vi "Destroy DAQmx Input Refs.vi"(8 "error in (no error)":errorcluster, 11 "DAQ":refnum<class "DAQ.lvclass">) -> (0 "error out":errorcluster, 3 "DAQ":refnum<class "DAQ.lvclass">)   [LabVIEW 2017, in "DAQ.lvclass"]
doc: "Developed by Kevin Thompson\nkevin@thompsonengineering.net\n\nCopyright 2018-2020\nThompson Engineering, LLC"
uses:
  DAQ.lvclass
  DAQ.lvclass/DAQ.ctl
  DataTypes/TD AI TaskIO.ctl
  DataTypes/TD DI TaskIO.ctl
  Accessors/Get DAQNodes Dict.vi
  Accessors/Get IO Nodes.vi
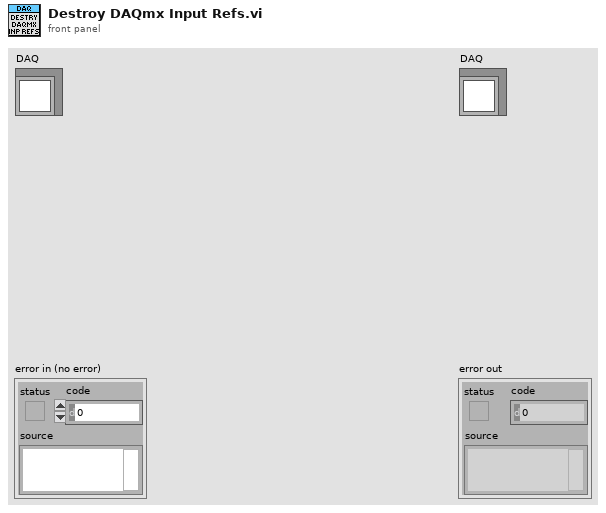
[diagram p1: front panel]
types:
  T1 = typedef "TD Dynamic CVT DVR--ref.ctl" = refnum<data-value>
  T2 = typedef "DAQ.lvclass/TD IO Config Definition--cluster.ctl" = cluster{"DI Config":T3, "DO Config":T6, "AI Config":T8, "AO Config":T14}
  T3 = typedef "DAQ.lvclass/TD DI Config--cluster.ctl" = cluster{"DI Tasks":T4[]}
  T4 = typedef "DAQ.lvclass/TD DI Task--cluster.ctl" = cluster{"DI TaskName":string, "DI Channels":T5[]}
  T5 = typedef "DAQ.lvclass/TD DI Channel--cluster.ctl" = cluster{"DevName":string, "IOName":string, "IOPath":string, "SchemName":string, "logic":enum16{"Lo", "Hi"}, "Index":i32}
  T6 = typedef "DAQ.lvclass/TD DO Config--cluster.ctl" = cluster{"DO Channels":T7[]}
  T7 = typedef "DAQ.lvclass/TD DO Channel--cluster.ctl" = cluster{"DevName":string, "IOName":string, "IOPath":string, "SchemName":string, "logic":enum16{"Lo", "Hi"}, "DAQmx Task":refnum<k21>}
  T8 = typedef "DAQ.lvclass/TD AI Config--cluster.ctl" = cluster{"AI Tasks":T9[]}
  T9 = typedef "DAQ.lvclass/TD AI Task--cluster.ctl" = cluster{"AI TaskName":string, "AI Channels":T10[]}
  T10 = typedef "DAQ.lvclass/TD AI Channel--cluster.ctl" = cluster{"DevName":string, "IOName":string, "IOPath":string, "SchemName":string, "MinValue":dbl, "MaxValue":dbl, "Terminal Configuration":i32, "Index":i32, "Conversion":T11, "AIType":T12, "Force Bridge":T13}
  T11 = typedef "DAQ.lvclass/TD DataValueConversion--cluster.ctl" = cluster{"MaxSignal":dbl, "MinSignal":dbl, "MaxEngUnit":dbl, "MinEngUnit":dbl, "ScaleOffset":dbl, "negate":bool}
  T12 = typedef "DAQ.lvclass/TD AI DAQ Type--enum.ctl" = enum16{"Voltage", "Current", "Strain Gage", "Force Bridge"}
  T13 = typedef "DAQ.lvclass/TD AI Force Bridge--cluster.ctl" = cluster{"bridge information":cluster{"bridge configuration":i32, "voltage excitation source":i32, "voltage excitation value":dbl, "nominal bridge resistance":dbl}, "scaling information":cluster{"first electrical value":dbl, "second electrical value":dbl, "electrical units":i32, "first physical value":dbl, "second physical value":dbl, "physical units":i32}}
  T14 = typedef "DAQ.lvclass/TD AO Config--cluster.ctl" = cluster{"AO Channels":T15[]}
  T15 = typedef "DAQ.lvclass/TD AO Channel--cluster.ctl" = cluster{"DevName":string, "IOName":string, "IOPath":string, "SchemName":string, "Vmin":dbl, "Vmax":dbl, "Conversion":T11, "DAQmx Task":refnum<k21>}
  T16 = typedef "DAQ.lvclass/TD AI TaskIO.ctl" = cluster{"AI TaskName":string, "IONames":string[], "DAQmx AI TaskRef":refnum<k21>}
  T17 = typedef "DAQ.lvclass/TD DI TaskIO.ctl" = cluster{"DI TaskName":string, "IONames":string[], "DAQmxDI TaskRef":refnum<k21>}
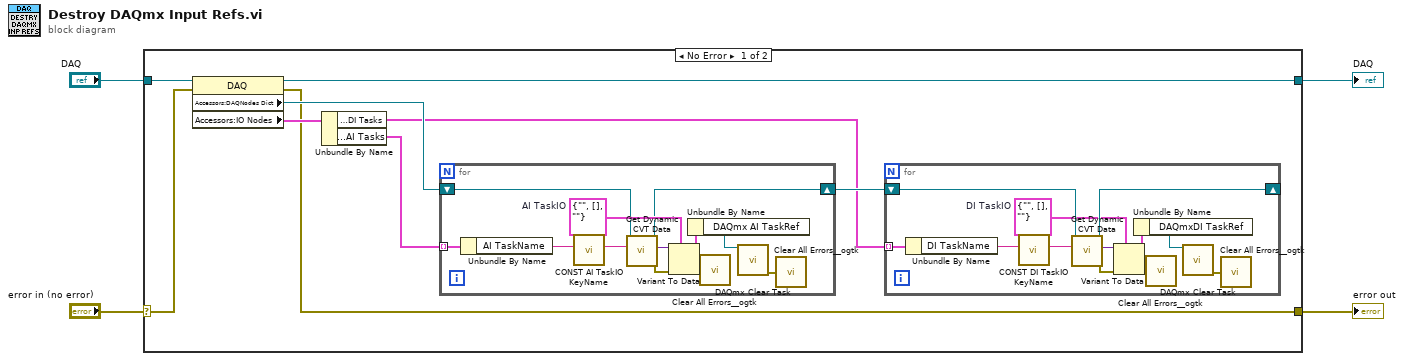
[diagram p0: block diagram]
diagram:
  n1 = case shown="No Error" "error in (no error)" {
    selector: "error in (no error)" -> [w6 w39]
    tunnel: [w5 w39] -> w3
    tunnel: [w12 w38] -> w1
    tunnel: "DAQ" -> [w13 w38]
    frame No Error {
      n2 = property class="DAQ"(reference=w13, error in=w6) -> (reference out=w12:refnum<class "DAQ.lvclass">, error out=w5:errorcluster, "Accessors:DAQNodes Dict"=w9:T1, "Accessors:IO Nodes"=w11:T2)
      n3 = Unbundle By Name(w11) -> ("DI Config.DI Tasks"=w7:T4[], "AI Config.AI Tasks"=w10:T9[])
      n4 = for {
        tunnel: w10 -> [w34] mode=indexing
        shift-right: [w27] -> w8
        shift-left: w9 -> [w28]
        w31 = T16 {"AI TaskName"="", "IONames"=[], "DAQmx AI TaskRef"=""}  # AI TaskIO
        n5 = Unbundle By Name(w34) -> ("AI TaskName"=w33:string)
        n6 = call "CONST AI TaskIO KeyName.vi"("AI TaskName"=w33) -> ("AI TaskIO (KeyName)"=w32:string)  [unwired: 10 in]
        n7 = call <vilib>:"Get Dynamic CVT Data.vi"("DataName"=w32, "dCVT DVR"=w28) -> ("error out"=w37:errorcluster, "value"=w36:variant, "dCVT DVR out"=w27:T1)  [unwired: 6 in, 1 out]
        n8 = Variant To Data(error in=w37, type=w31, Variant=w36) -> (data=w30:T16, error out=w26:errorcluster)
        n9 = Unbundle By Name(w30) -> ("DAQmx AI TaskRef"=w29:refnum<k21>)
        n10 = call <userlib>:"Clear All Errors__ogtk.vi"("Error In"=w26) -> ()  [unwired: 3 in, 1 out]
        n11 = call <vilib>:"DAQmx Clear Task.vi"("task in"=w29) -> ("error out"=w35:errorcluster)  [unwired: 14 in]
        n12 = call <userlib>:"Clear All Errors__ogtk.vi"("Error In"=w35) -> ()  [unwired: 3 in, 1 out]
      }
      n13 = for {
        tunnel: w7 -> [w22] mode=indexing
        shift-right: [w18] -> _
        shift-left: w8 -> [w19]
        w17 = T17 {"DI TaskName"="", "IONames"=[], "DAQmxDI TaskRef"=""}  # DI TaskIO
        n14 = Unbundle By Name(w22) -> ("DI TaskName"=w16:string)
        n15 = call "CONST DI TaskIO KeyName.vi"("DI TaskName"=w16) -> ("DI TaskIO (KeyName)"=w15:string)  [unwired: 10 in]
        n16 = call <vilib>:"Get Dynamic CVT Data.vi"("DataName"=w15, "dCVT DVR"=w19) -> ("error out"=w25:errorcluster, "value"=w24:variant, "dCVT DVR out"=w18:T1)  [unwired: 6 in, 1 out]
        n17 = Variant To Data(error in=w25, type=w17, Variant=w24) -> (data=w21:T17, error out=w14:errorcluster)
        n18 = Unbundle By Name(w21) -> ("DAQmxDI TaskRef"=w20:refnum<k21>)
        n19 = call <userlib>:"Clear All Errors__ogtk.vi"("Error In"=w14) -> ()  [unwired: 3 in, 1 out]
        n20 = call <vilib>:"DAQmx Clear Task.vi"("task in"=w20) -> ("error out"=w23:errorcluster)  [unwired: 14 in]
        n21 = call <userlib>:"Clear All Errors__ogtk.vi"("Error In"=w23) -> ()  [unwired: 3 in, 1 out]
      }
    }
    frame Error {
    }
  }
  "error out" <- w3
  "DAQ" <- w1
